vi "Scope Conf Trigger.vi"(8 "error in (no error)":errorcluster, 11 "Actor_Scope in":refnum<class "Actor_Scope.lvclass">) -> (0 "error out":errorcluster, 3 "Actor_Scope out":refnum<class "Actor_Scope.lvclass">)   [LabVIEW 2020, in "Actor_Scope.lvlib" / "Actor_Scope.lvclass"]
uses:
  Actor_Scope.lvclass
  Actor_Scope.lvclass/Actor_Scope.ctl
  <instrlib>/Agilent 8000 Series/Public/Configure/Configure Trigger (Edge).vi
  <instrlib>/Agilent 8000 Series/Agilent 8000 Series.lvlib
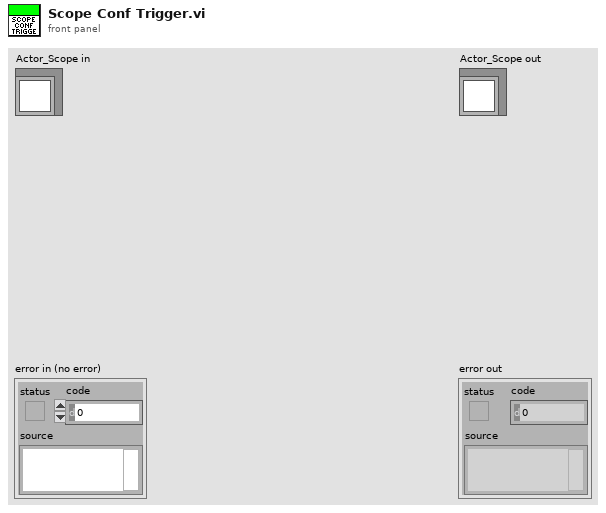
[diagram p1: front panel]
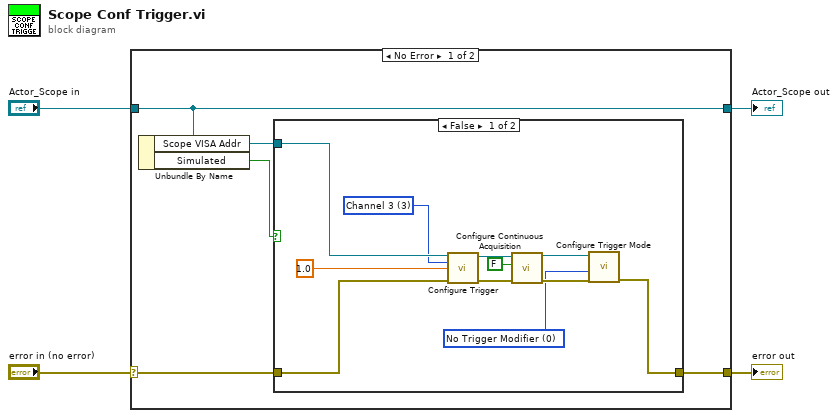
[diagram p0: block diagram]
diagram:
  n1 = case shown="No Error" "error in (no error)" {
    selector: "error in (no error)" -> [w5 w23]
    tunnel: [w8 w23] -> w3
    tunnel: [w9 w22] -> w1
    tunnel: "Actor_Scope in" -> [w9 w22]
    frame No Error {
      n2 = Unbundle By Name(w9) -> ("Scope VISA Addr"=w7:refnum<visa-resource-name>, "Simulated"=w6:bool)
      n3 = case shown="False" w6 {
        tunnel: [w16 w21] -> w8
        tunnel: w7 -> [w15 _]
        tunnel: w5 -> [w12 w21]
        frame False {
          w11 = 3 items=["Channel 1"=1, "Channel 2"=2, "Channel 3"=3, "Channel 4"=4, "Digital 0"=13, "Digital 1"=14, "Digital 2"=15, "Digital 3"=16, "Digital 4"=17, "Digital 5"=18, "Digital 6"=19, "Digital 7"=20, "Digital 8"=21, "Digital 9"=22, "Digital 10"=23, "Digital 11"=24, "Digital 12"=25, "Digital 13"=26, "Digital 14"=27, "Digital 15"=28, "Aux"=29, "Line"=30] ("Trigger Source (1: Channel 1)")
          w17 = u16 0 items=["No Trigger Modifier", "Auto"] ("Trigger Modifier (0: No Trigger Modifier)")
          n4 = call-poly <instrlib>:"Configure Trigger.vi"("VISA resource name"=w15, "Trigger Source (1: Channel 1)"=w11, "Trigger Level (0.0 V)"=1.0, "error in (no error)"=w12) -> ("VISA resource name out"=w14:refnum<visa-resource-name>, "error out"=w13:errorcluster)  [unwired: 10 in]
          n5 = call <instrlib>:"Configure Continuous Acquisition.vi"("error in (no error)"=w13, "Enable Continuous Acquisition Mode (T:Enable)"=FALSE, "VISA resource name"=w14) -> ("error out"=w18:errorcluster, "VISA resource name out"=w19:refnum<visa-resource-name>)  [unwired: 7 in]
          n6 = call <instrlib>:"Configure Trigger Mode.vi"("error in (no error)"=w18, "Trigger Modifier (0: No Trigger Modifier)"=w17, "VISA resource name"=w19) -> ("error out"=w16:errorcluster)  [unwired: 7 in, 1 out]
        }
        frame True {
        }
      }
    }
    frame Error {
    }
  }
  "error out" <- w3
  "Actor_Scope out" <- w1
